vi "Configure Idle.vi"(8 "error in (no error)":errorcluster, 11 "FGen PXI Base CFG in":refnum<class "FGen PXI Base CFG.lvclass">) -> (0 "error out":errorcluster, 3 "FGen PXI Base CFG out":refnum<class "FGen PXI Base CFG.lvclass">)   [LabVIEW 2023, in "FGen PXI Base CFG.lvlib" / "FGen PXI Base CFG.lvclass"]
uses:
  FGen PXI Base CFG.lvclass
  7d5647a1-ee57-477e-af02-dfb71140fe97.vi
  <vilib>/ErrorRing/Error Ring.xnode
  <vilib>/Utility/error.llb/Error Cluster From Error Code.vi
  Configuration JSON Base/CFG JSON Base.lvclass
  D:/git/HAL/HAL GOOP4/FGen/FGen Base CFG/FGen Base CFG.lvclass
  D:/git/HAL/HAL GOOP4/Configuration JSON Base/CFG JSON Base.lvclass
  D:/git/HAL/HAL GOOP4/Interfaces/IConfigure/IConfigure.lvclass
  D:/git/HAL/HAL GOOP4/FGen/FGen PXI/FGen PXI Base CFG/FGen PXI Base CFG.lvclass
panel:
  out "Output:Advanced:Idle Behavior":i32(ring)=400 items=["Hold Last Value"=400, "Jump To Value"=401]
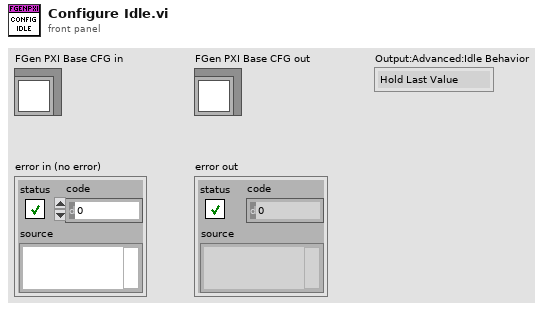
[diagram p1: front panel]
types:
  T1 = cluster{"Idle Behavior":string, "Idle Value":i32}
  T2 = typedef "LVStringsAndValuesArrayTypeDef_I32.ctl" = cluster{"String":string, "Value":i32}[]
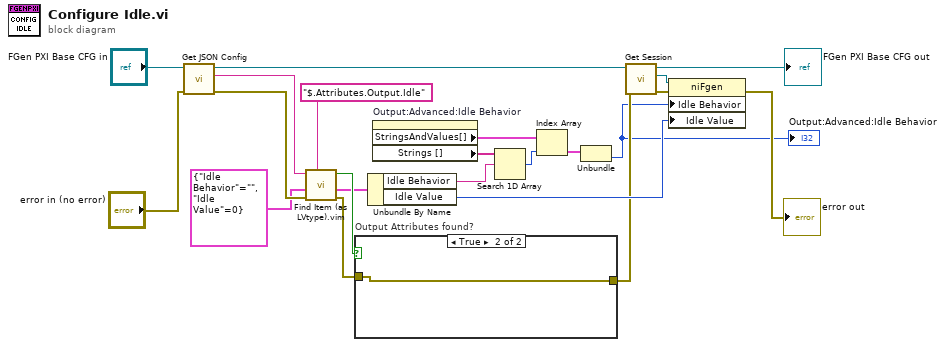
[diagram p0: block diagram]
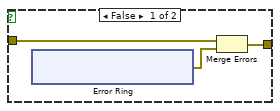
[diagram p2: hidden frame]
diagram:
  n1 = call "Get JSON Config.vi"("error in (no error)"="error in (no error)", "CFG Base in"="FGen PXI Base CFG in") -> ("error out"=w14:errorcluster, "<JSON>Config>"=w15:string, "CFG Base out"=w17:refnum<class "FGen PXI Base CFG.lvclass">)  [unwired: 7 in]
  n2 = call "Find Item (as LVtype).vim"("$Path or Item Name"="$.Attributes.Output.Idle", "error in (no error)"=w14, "Data Type and Default Value"=T1 {"Idle Behavior"="", "Idle Value"=0}, "JSON"=w15) -> ("error out"=w11:errorcluster, "Data"=w10:T1, "Found"=w12:bool)  [unwired: 4 in, 1 out]
  n3 = case "Output Attributes found?" shown="True" w12 {
    tunnel: w11 -> [w25 w31]
    tunnel: [w23 w31] -> w4
    frame False {
      n4 = xnode "Error Ring"() -> ("error out"=w24:errorcluster)
      n5 = Merge Errors(w25, w24) -> (w23:errorcluster)
    }
    frame True {
    }
  }
  n6 = Unbundle By Name(w10) -> ("Idle Behavior"=w9:string, "Idle Value"=w5:i32)
  n7 = property on="Output:Advanced:Idle Behavior" class="Ring (strict)"() -> ("StringsAndValues[]"=w8:T2, "Strings []"=w19:string[])  [unwired: 2 in, 2 out]
  n8 = Search 1D Array(1D array=w19, element=w9) -> (index of element=w3:i32)  [unwired: 1 in]
  n9 = Index Array(array=w8, index=w3) -> (element=w7:cluster{"String":string, "Value":i32})
  n10 = Unbundle(w7) -> ("Value"=w1:i32)  [unwired: 1 out]
  "Output:Advanced:Idle Behavior" <- w1
  n11 = call "Get Session.vi"("error in (no error)"=w4, "FGen PXI Base CFG in"=w17) -> ("error out"=w6:errorcluster, "Session"=w20:refnum<k15>, "FGen PXI Base CFG out"=→"FGen PXI Base CFG out":refnum<class "FGen PXI Base CFG.lvclass">)  [unwired: 7 in]
  n12 = property class="niFgen"(reference=w20, error in=w6, "Idle Behavior"=w1, "Idle Value"=w5) -> (error out=→"error out":errorcluster)  [unwired: 1 out]
